vi "GetEventAppliedStaticForcesField.vi"(10 "Event Data":string, 11 "Cluster in":refnum<vi>) -> (3 "Array":string[](array[string]))   [LabVIEW 2016]
uses:
  SALLV_m1m3/DataTypes/logevent_AppliedStaticForces.ctl
  SALLV_m1m3/SALLV_m1m3.lvlib
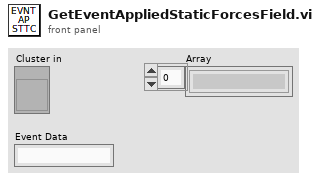
[diagram p1: front panel]
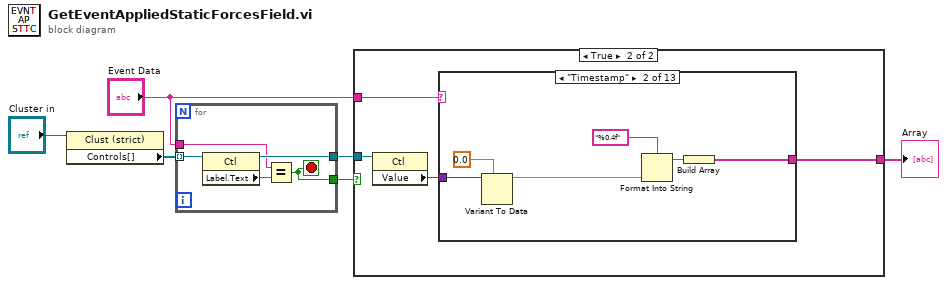
[diagram p0: block diagram]
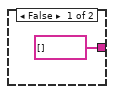
[diagram p2: hidden frame]
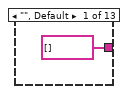
[diagram p3: hidden frame]
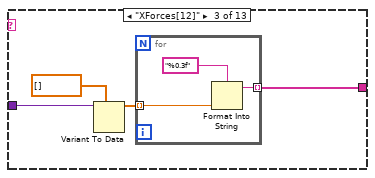
[diagram p4: hidden frame]
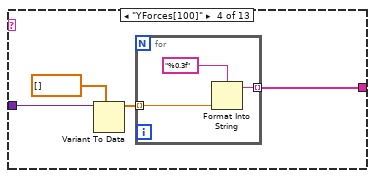
[diagram p5: hidden frame]
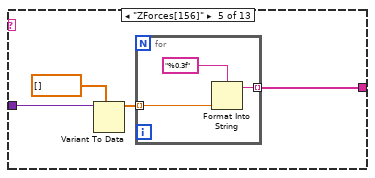
[diagram p6: hidden frame]
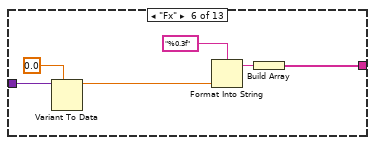
[diagram p7: hidden frame]
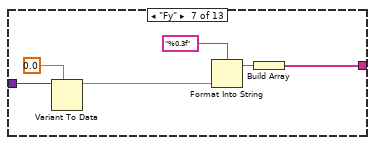
[diagram p8: hidden frame]
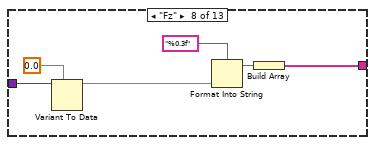
[diagram p9: hidden frame]
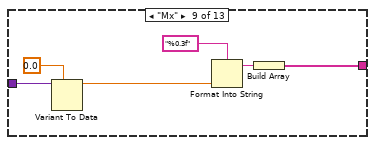
[diagram p10: hidden frame]
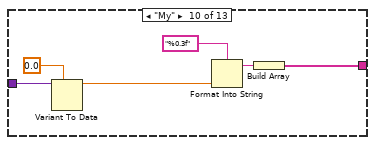
[diagram p11: hidden frame]
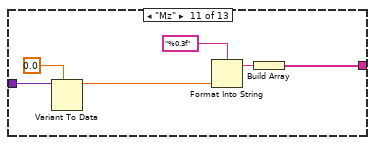
[diagram p12: hidden frame]
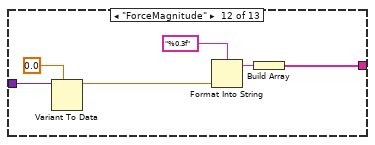
[diagram p13: hidden frame]
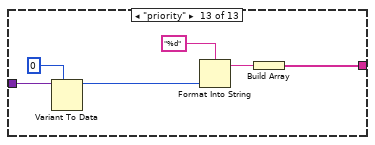
[diagram p14: hidden frame]
diagram:
  n1 = property on="Property Node" class="Clust (strict)"(reference="Cluster in") -> ("Controls[]"=w6:refnum<vi>[])  [unwired: 1 in, 2 out]
  n2 = for {
    tunnel: w6 -> [w11] mode=indexing
    tunnel: [w10] -> w4
    tunnel: "Event Data" -> [w8]
    tunnel: [w7] -> w5
    stop <- w7 stop-if-true
    n3 = property on="Property Node" class="Ctl"(reference=w11) -> (reference out=w10:refnum<vi>, "Label.Text"=w9:string)  [unwired: 1 in, 1 out]
    n4 = Equal?(x=w8, y=w9) -> (x = y?=w7:bool)
  }
  n5 = case shown="True" w5 {
    tunnel: "Event Data" -> [_ w16]
    tunnel: w4 -> [_ w15]
    tunnel: [string[] [] w13] -> w2
    frame False {
    }
    frame True {
      n6 = property on="Property Node" class="Ctl"(reference=w15) -> ("Value"=w14:variant)  [unwired: 1 in, 2 out]
      n7 = case shown="\"Timestamp\"" w16 {
        tunnel: [string[] [] w21 w24 w31 w38 w48 w54 w60 w66 w72 w78 w84 w90] -> w13
        tunnel: w14 -> [_ w19 w27 w34 w41 w46 w52 w58 w64 w70 w76 w82 w88]
        frame "", Default {
        }
        frame "Timestamp" {
          n8 = Variant To Data(type=0.0, Variant=w19) -> (data=w20:dbl)  [unwired: 1 in, 1 out]
          n9 = Format Into String(format string="%0.4f", w20) -> (resulting string=w22:string)  [unwired: 2 in, 1 out]
          n10 = Build Array(w22) -> (w21:string[])
        }
        frame "XForces[12]" {
          n11 = Variant To Data(type=sgl[] [], Variant=w27) -> (data=w25:sgl[])  [unwired: 1 in, 1 out]
          n12 = for {
            tunnel: w25 -> [w29] mode=indexing
            tunnel: [w28] -> w24 mode=indexing
            n13 = Format Into String(format string="%0.3f", w29) -> (resulting string=w28:string)  [unwired: 2 in, 1 out]
          }
        }
        frame "YForces[100]" {
          n14 = Variant To Data(type=sgl[] [], Variant=w34) -> (data=w32:sgl[])  [unwired: 1 in, 1 out]
          n15 = for {
            tunnel: w32 -> [w36] mode=indexing
            tunnel: [w35] -> w31 mode=indexing
            n16 = Format Into String(format string="%0.3f", w36) -> (resulting string=w35:string)  [unwired: 2 in, 1 out]
          }
        }
        frame "ZForces[156]" {
          n17 = Variant To Data(type=sgl[] [], Variant=w41) -> (data=w39:sgl[])  [unwired: 1 in, 1 out]
          n18 = for {
            tunnel: w39 -> [w43] mode=indexing
            tunnel: [w42] -> w38 mode=indexing
            n19 = Format Into String(format string="%0.3f", w43) -> (resulting string=w42:string)  [unwired: 2 in, 1 out]
          }
        }
        frame "Fx" {
          n20 = Variant To Data(type=0.0, Variant=w46) -> (data=w47:dbl)  [unwired: 1 in, 1 out]
          n21 = Format Into String(format string="%0.3f", w47) -> (resulting string=w49:string)  [unwired: 2 in, 1 out]
          n22 = Build Array(w49) -> (w48:string[])
        }
        frame "Fy" {
          n23 = Variant To Data(type=0.0, Variant=w52) -> (data=w53:dbl)  [unwired: 1 in, 1 out]
          n24 = Format Into String(format string="%0.3f", w53) -> (resulting string=w55:string)  [unwired: 2 in, 1 out]
          n25 = Build Array(w55) -> (w54:string[])
        }
        frame "Fz" {
          n26 = Variant To Data(type=0.0, Variant=w58) -> (data=w59:dbl)  [unwired: 1 in, 1 out]
          n27 = Format Into String(format string="%0.3f", w59) -> (resulting string=w61:string)  [unwired: 2 in, 1 out]
          n28 = Build Array(w61) -> (w60:string[])
        }
        frame "Mx" {
          n29 = Variant To Data(type=0.0, Variant=w64) -> (data=w65:dbl)  [unwired: 1 in, 1 out]
          n30 = Format Into String(format string="%0.3f", w65) -> (resulting string=w67:string)  [unwired: 2 in, 1 out]
          n31 = Build Array(w67) -> (w66:string[])
        }
        frame "My" {
          n32 = Variant To Data(type=0.0, Variant=w70) -> (data=w71:dbl)  [unwired: 1 in, 1 out]
          n33 = Format Into String(format string="%0.3f", w71) -> (resulting string=w73:string)  [unwired: 2 in, 1 out]
          n34 = Build Array(w73) -> (w72:string[])
        }
        frame "Mz" {
          n35 = Variant To Data(type=0.0, Variant=w76) -> (data=w77:dbl)  [unwired: 1 in, 1 out]
          n36 = Format Into String(format string="%0.3f", w77) -> (resulting string=w79:string)  [unwired: 2 in, 1 out]
          n37 = Build Array(w79) -> (w78:string[])
        }
        frame "ForceMagnitude" {
          n38 = Variant To Data(type=0.0, Variant=w82) -> (data=w83:dbl)  [unwired: 1 in, 1 out]
          n39 = Format Into String(format string="%0.3f", w83) -> (resulting string=w85:string)  [unwired: 2 in, 1 out]
          n40 = Build Array(w85) -> (w84:string[])
        }
        frame "priority" {
          n41 = Variant To Data(type=0, Variant=w88) -> (data=w89:i32)  [unwired: 1 in, 1 out]
          n42 = Format Into String(format string="%d", w89) -> (resulting string=w91:string)  [unwired: 2 in, 1 out]
          n43 = Build Array(w91) -> (w90:string[])
        }
      }
    }
  }
  "Array" <- w2
